vi "改变图像格式.vi"() -> ()   [LabVIEW 2018]
panel:
  out "error out":errorcluster
  out "Image":T1(plugin-control)
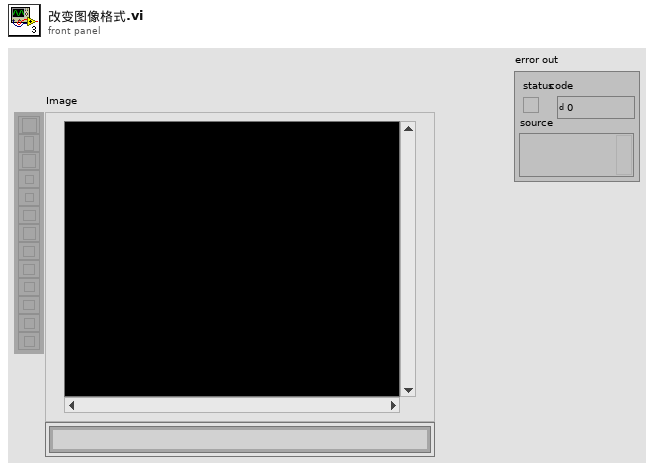
[diagram p1: front panel]
types:
  T1 = typedef "IMAQ Image.ctl" = refnum<image>
  T2 = typedef "Image Type" = u32
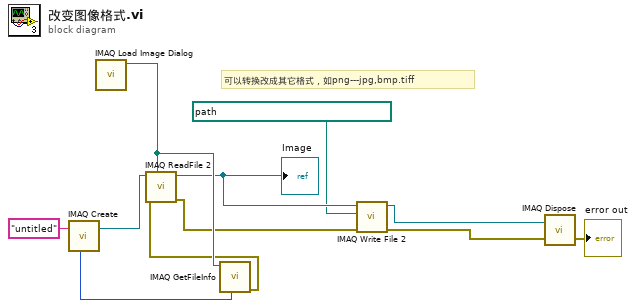
[diagram p0: block diagram]
diagram:
  # "可以转换改成其它格式，如png---jpg,bmp.tiff"
  n1 = call "IMAQ Load Image Dialog"() -> ("Path"=w10:path)  [unwired: 9 in, 2 out]
  n2 = call "IMAQ GetFileInfo"("File Path"=w10) -> ("error out"=w7:errorcluster, "Image Type"=w11:T2)  [unwired: 4 in, 5 out]
  n3 = call "IMAQ Create"("Image Name"="untitled", "Image Type"=w11) -> ("New Image"=w9:T1)  [unwired: 3 in, 1 out]
  n4 = call "IMAQ ReadFile 2"("File Path"=w10, "error in (no error)"=w7, "Image"=w9) -> ("error out"=w3:errorcluster, "Image Out"=w4:T1)  [unwired: 4 in, 3 out]
  "Image" <- w4
  n5 = call-poly "IMAQ Write File 2"("error in (no error)"=w3, "File Path"=path "D:/Labviewprogram/视觉/11.jpg", "Image"=w4) -> ("error out"=w5:errorcluster, "Image Out (duplicate)"=w6:T1)  [unwired: 7 in]
  n6 = call "IMAQ Dispose"("Image"=w6, "error in (no error)"=w5) -> ("error out"=→"error out":errorcluster)  [unwired: 4 in]
